vi "GetInputShapeDim.vi"(8 "error in (no error)":errorcluster, 9 "dimIndex":i32, 10 "inputIndex":i32, 11 "session id in":i32) -> (0 "error out":errorcluster, 2 "InputShapeDim":i64, 3 "session id out":i32)   [LabVIEW 2017, in "libonnx_wrapper.lvlib"]
doc: "/**\n * @brief Получить значение конкретной размерности входного тензора\n * \n * Возвращает размер тензора по указанному измерению.\n * Например, для shape [1, 3, 224, 224]:\n * - dimIndex=0 вернёт 1 (батч)\n * - dimIndex=1 вернёт 3 (каналы)\n * - dimIndex=2 вернёт 224 (высота)\n * - dimIndex=3 вернёт 224 (ширина)\n * \n * @param sessionId [IN] ID сессии\n * @param inputIndex [IN] Индекс входа (0-based)\n * @param dimIndex [IN] Индекс размерности (0-based, от 0 до GetInputShapeDimCount-1)\n * \n * @return int64: Значение размерности (положительное число)\n * @return int64: -1 если сессия не найдена или индексы неверны\n */\nint64_t GetInputShapeDim(int sessionId, int inputIndex, int dimIndex);"
uses:
  libonnx_wrapper.lvlib
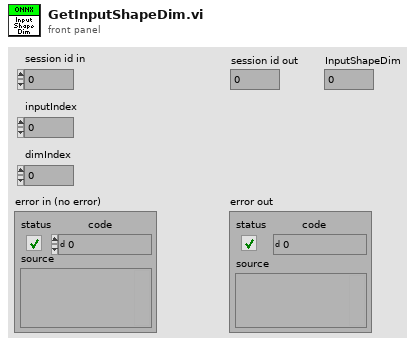
[diagram p1: front panel]
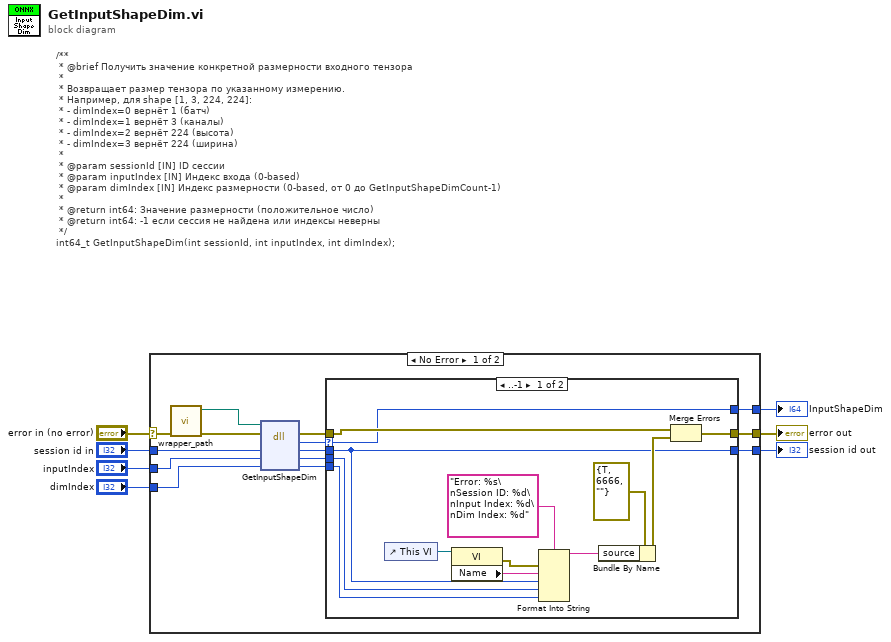
[diagram p0: block diagram]
diagram:
  # "/**\n * @brief Получить значение конкретной размерности входного тензора\n * \n * Возвращает размер тензора по указанному измерению.\n * Например, для shape [1, 3, 224, 224]:\n * - dimIndex=0 вернёт 1 (батч)\n * - dimIndex=1 вернёт 3 (каналы)\n * - dimIndex=2 вернёт 224 (высота)\n * - dimIndex=3 вернёт 224 (ширина)\n * \n * @param sessionId [IN] ID сессии\n * @param inputIndex [IN] Индекс входа (0-based)\n * @param dimIndex [IN] Индекс размерности (0-based, от 0 до GetInputShapeDimCount-1)\n * \n * @return int64: Значение размерности (положительное число)\n * @return int64: -1 если сессия не найдена или индексы неверны\n */\nint64_t GetInputShapeDim(int sessionId, int inputIndex, int dimIndex);"
  n1 = case shown="No Error" "error in (no error)" {
    selector: "error in (no error)" -> [w8 w39]
    tunnel: "inputIndex" -> [w21 _]
    tunnel: "session id in" -> [w19 w38]
    tunnel: "dimIndex" -> [w17 _]
    tunnel: [w13 w39] -> w4
    tunnel: [w12 w38] -> w3
    tunnel: [w11 _] -> w2
    frame No Error {
      n2 = call "wrapper_path.vi"("error in (no error)"=w8) -> ("error out"=w18:errorcluster, "wrapper path"=w20:path)  [unwired: 9 in]
      n3 = dll-call lib="home/ivan/LabVIEWData/ONNX/Test/libonnx_wrapper/unix64/libonnx_wrapper.so" fn="GetInputShapeDim"(path in=w20, error in=w18, "sessionId"=w19, "inputIndex"=w21, "dimIndex"=w17) -> (error out=w16:errorcluster, "return"=w15:i64, "sessionId"=w14:i32, "inputIndex"=w10:i32, "dimIndex"=w9:i32)  [unwired: 1 in, 1 out]
      n4 = case shown="..-1" w15 {
        selector: w15 -> [w23 w35]
        tunnel: w16 -> [w25 w37]
        tunnel: [w26 w37] -> w13
        tunnel: w14 -> [w27 w36]
        tunnel: [w27 w36] -> w12
        tunnel: w10 -> [w24 _]
        tunnel: [w23 w35] -> w11
        tunnel: w9 -> [w22 _]
        frame ..-1 {
          n5 = control-ref of="This VI"() -> (w31:refnum<vi>)
          n6 = property class="VI"(reference=w31) -> (error out=w28:errorcluster, "Name"=w30:string)  [unwired: 1 in, 1 out]
          n7 = Format Into String(format string="Error: %s\nSession ID: %d\nInput Index: %d\nDim Index: %d", error in=w28, w30, w27, w24, w22) -> (resulting string=w32:string)  [unwired: 1 in, 1 out]
          n8 = Bundle By Name(cluster=errorcluster {"status"=TRUE, "code"=6666, "source"=""} ("error out"), "source"=w32) -> (w33:errorcluster)
          n9 = Merge Errors(w25, w33) -> (w26:errorcluster)
        }
        frame 0.. {
        }
      }
    }
    frame Error {
    }
  }
  "error out" <- w4
  "session id out" <- w3
  "InputShapeDim" <- w2
